vi "AutoAlign_P541.vi"() -> ()   [LabVIEW 2011]
uses:
  Controls/GraphNotifier2D.ctl
  Controls/StageStates.ctl
  <vilib>/LabVIEW Interface for Arduino/LabVIEW Interface for Arduino.lvlib
panel:
  out "Current Step":i32
  in  "Done":bool
  in  "Repeat":bool
  in  "Start":bool
  out "Cursor Position":dbl=40.46
  in  "InitialStep":dbl=-0.5
  in  "StepSize":dbl=0.03
  in  "Number Of Steps":i32=45
  out "Intensity Graph":sgl[][](graph)=[[1726.0, 1806.0, 1623.0, 1740.0, 1902.0, 2025.0, 2061.0, 2397.0, 1982.0, 2142.0, 1921.0, 1825.0, 1807.0, 1676.0, 1719.0], [1834.0, 1961.0, 1598.0, 2017.0, 2102.0, 2328.0, 2583.0, 2454.0, 2515.0, 2699.0, 2220.0, 2038.0, 1897.0, 1896.0, 1808.0], [1796.0, 1929.0, 2014.0, 2227.0, 2672.0, 3226.0, 3334.0, 3386.0, 3268.0, 2996.0, 2332.0, 2163.0, 1901.0, 1735.0, 1698.0], [1808.0, 2338.0, 2431.0, 2752.0, 3453.0, 4017.0, 4563.0, 4369.0, 4047.0, 3273.0, 2724.0, 2242.0, 2046.0, 1830.0, 1856.0], [1912.0, 2124.0, 3081.0, 2979.0, 5386.0, 11058.0, 13706.0, 11119.0, 6549.0, 3853.0, 2769.0, 2421.0, 1921.0, 1945.0, 1667.0], [1802.0, 2329.0, 2974.0, 5101.0, 13243.0, 29557.0, 37323.0, 29866.0, 11701.0, 4217.0, 2995.0, 2488.0, 2124.0, 2138.0, 1748.0], [1855.0, 2667.0, 2858.0, 6518.0, 22689.0, 47134.0, 57757.0, 40932.0, 16892.0, 4794.0, 2975.0, 2648.0, 2316.0, 1940.0, 2196.0], [1840.0, 2513.0, 2969.0, 6113.0, 20925.0, 44575.0, 52306.0, 35893.0, 13438.0, 3959.0, 2980.0, 2333.0, 2128.0, 1717.0, 1820.0], [1975.0, 2578.0, 2513.0, 4337.0, 10762.0, 22714.0, 27719.0, 17796.0, 6495.0, 3198.0, 2732.0, 2148.0, 1973.0, 1982.0, 1689.0], [1678.0, 2147.0, 2574.0, 2995.0, 4337.0, 7306.0, 8045.0, 5820.0, 3423.0, 2628.0, 2656.0, 2059.0, 2116.0, 1972.0, 1626.0], [1892.0, 2079.0, 2546.0, 2756.0, 2841.0, 3166.0, 3141.0, 2947.0, 2684.0, 2415.0, 1923.0, 1806.0, 2081.0, 1695.0, 1756.0], [1617.0, 1885.0, 1958.0, 2510.0, 2675.0, 2479.0, 2435.0, 2624.0, 2645.0, 2107.0, 1819.0, 2019.0, 1839.0, 1623.0, 1670.0], [1609.0, 1896.0, 1887.0, 1962.0, 2214.0, 2352.0, 2290.0, 2047.0, 1815.0, 2022.0, 1883.0, 1801.0, 1521.0, 1615.0, 1723.0], [1697.0, 1808.0, 1977.0, 1969.0, 2042.0, 1988.0, 2305.0, 2063.0, 1959.0, 1814.0, 1844.0, 1590.0, 1578.0, 1755.0, 1573.0], [1645.0, 1684.0, 1821.0, 1765.0, 1973.0, 1906.0, 2005.0, 1822.0, 1736.0, 1850.0, 1649.0, 1802.0, 1476.0, 1658.0, 1637.0]]
  in  "Quit":bool
  out "Sample":cluster{"X":dbl, "Y":dbl}[](graph)
  in  "Accumulations":i32=10
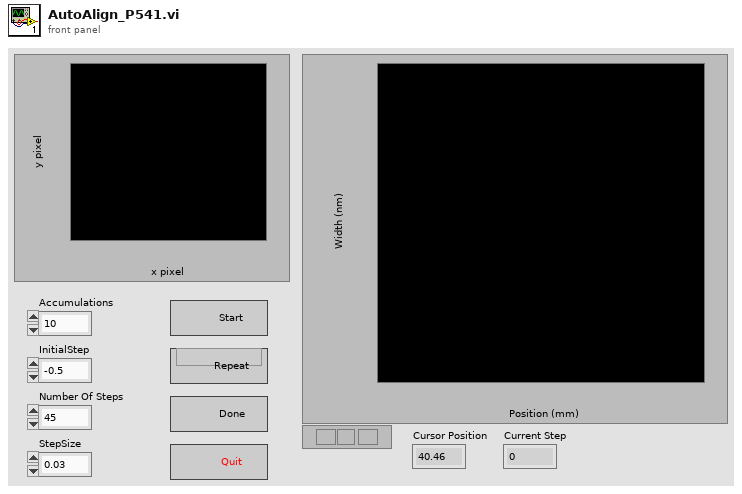
[diagram p1: front panel]
types:
  T1 = typedef "GraphNotifier2D.ctl" = cluster{"Xpos":i32, "Ypos":i32, "subarray":sgl[][], "Intensity":sgl}
  T2 = typedef "LabVIEW Interface for Arduino.lvlib/Arduino Resource.ctl" = cluster{"VISA resource":refnum<visa-resource-name>, "Board Type":T3, "Connection Type":enum8{"USB / Serial"}, "Bytes Per Packet (15)":u8}
  T3 = typedef "LabVIEW Interface for Arduino.lvlib/Board Type.ctl" = enum16{"Uno", "Dimuelanove w/Atmega 328", "Mega 2560"}
  T4 = typedef "StageStates.ctl" = enum16{"POSITION", "MVR", "MOVE", "HALT", "ONTARGET", "ERROR", "EXIT", "HOME", "ZEROPOS", "NANOPOS", "QUIT", "ANALOG"}
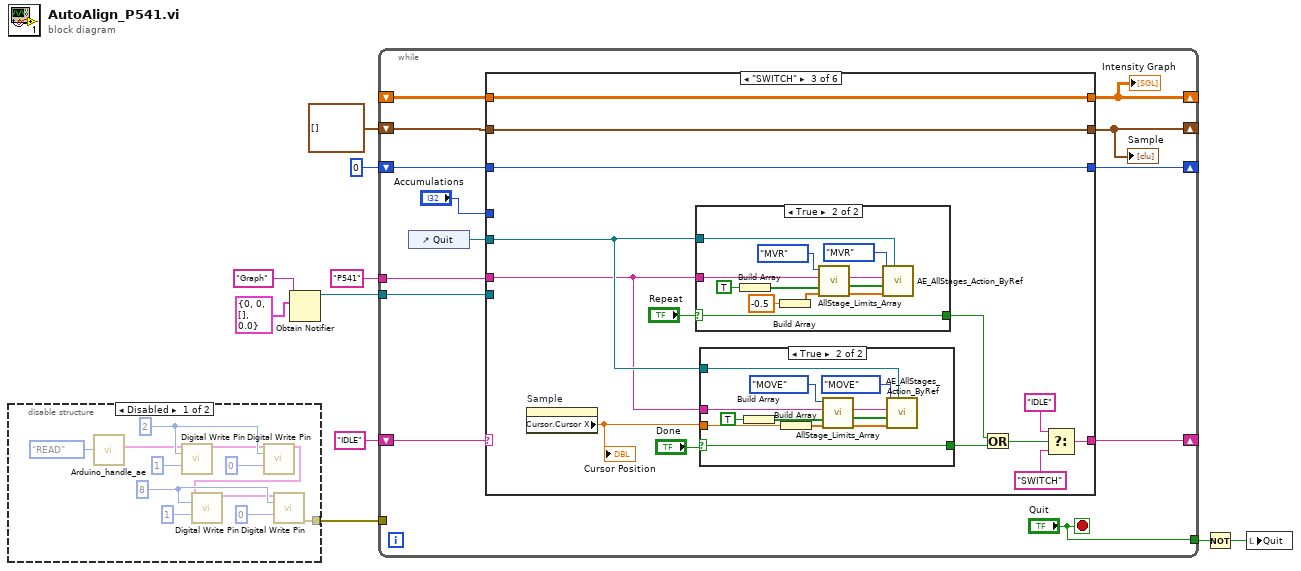
[diagram p0: block diagram]
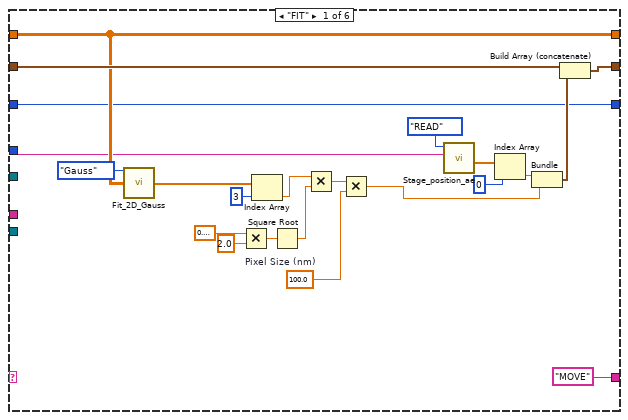
[diagram p3: hidden frame]
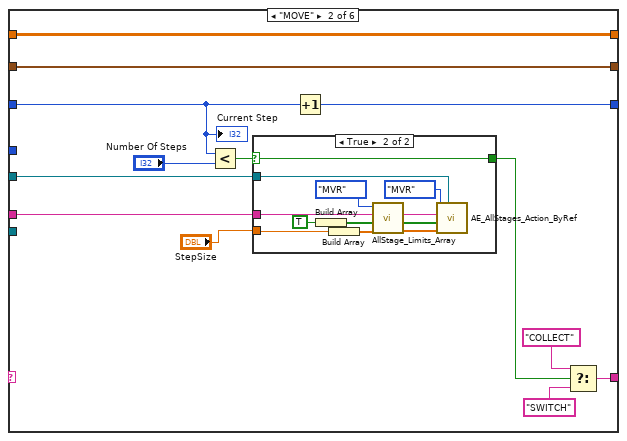
[diagram p4: hidden frame]
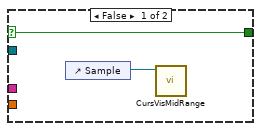
[diagram p5: hidden frame]
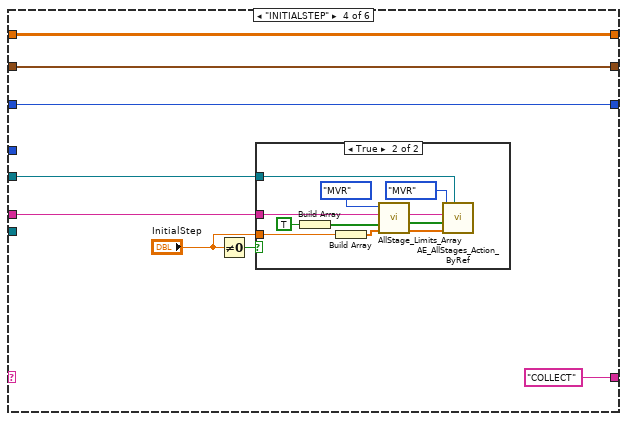
[diagram p8: hidden frame]
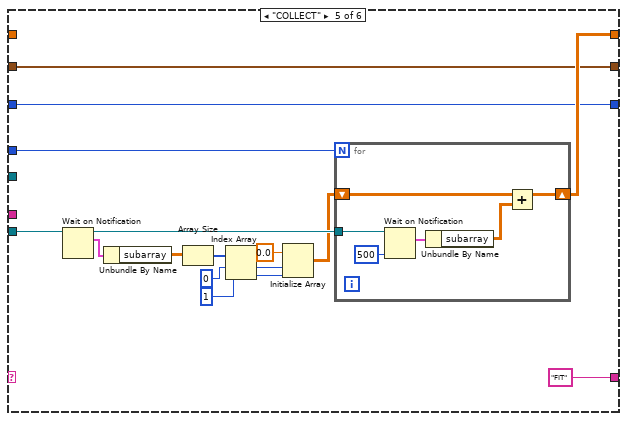
[diagram p10: hidden frame]
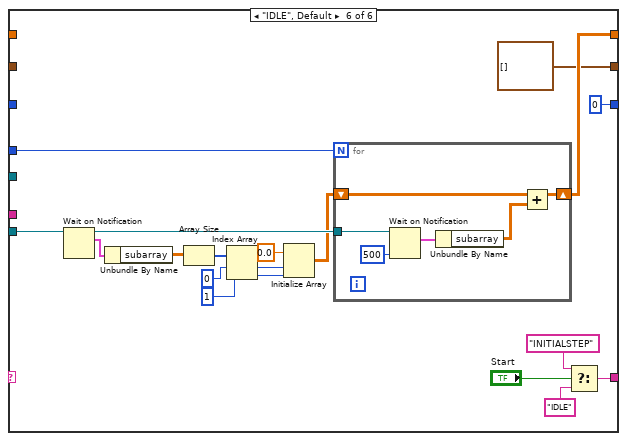
[diagram p11: hidden frame]
diagram:
  n1 = disable-structure shown="Disabled" {
    disable-tunnel: [w11 _] -> w6
    frame Disabled {
      w22 = u8 8 ("Digital I/O Pin (0)")
      w17 = u8 2 ("Digital I/O Pin (0)")
      n2 = call "Arduino_handle_ae.vi"("Enum"=enum16{"WRITE", "READ"}."READ") -> ("Arduino Resource Out"=w16:T2)  [unwired: 10 in]
      n3 = call <vilib>:"Digital Write Pin.vi"("Arduino Resource"=w16, "Digital I/O Pin (0)"=w17, "Value (0)"=u8 1) -> ("Arduino Resource"=w12:T2)  [unwired: 11 in, 1 out]
      n4 = call <vilib>:"Digital Write Pin.vi"("Arduino Resource"=w12, "Digital I/O Pin (0)"=w17, "Value (0)"=u8 0) -> ("Arduino Resource"=w21:T2)  [unwired: 11 in, 1 out]
      n5 = call <vilib>:"Digital Write Pin.vi"("Arduino Resource"=w21, "Digital I/O Pin (0)"=w22, "Value (0)"=u8 1) -> ("Arduino Resource"=w20:T2)  [unwired: 11 in, 1 out]
      n6 = call <vilib>:"Digital Write Pin.vi"("Arduino Resource"=w20, "Digital I/O Pin (0)"=w22, "Value (0)"=u8 0) -> ("error out"=w11:errorcluster)  [unwired: 11 in, 1 out]
    }
    frame Enabled {
    }
  }
  n7 = Obtain Notifier(name (unnamed)="Graph", notification data type=T1 {"Xpos"=0, "Ypos"=0, "subarray"=[], "Intensity"=0.0}) -> (notifier out=w3:refnum<notifier>)  [unwired: 2 in, 2 out]
  n8 = while {
    shift-right: [w33] -> _
    shift-left: _ -> [w35]
    shift-right: [w34] -> _
    shift-left: cluster{"x":dbl, "y":dbl}[] [] ("XY chart data") -> [w24]
    shift-right: [w32] -> _
    shift-left: "IDLE" -> [w28]
    shift-right: [w30] -> _
    shift-left: 0 ("NumberOfSteps 2") -> [w31]
    tunnel: w3 -> [w27]
    tunnel: "P541" ("StageID") -> [w25]
    tunnel: w6 -> [_]
    tunnel: ["Quit"] -> w2
    stop <- "Quit" stop-if-true
    n9 = control-ref of="Quit"() -> (w29:refnum<vi>)
    n10 = case shown="\"SWITCH\"" w28 {
      tunnel: [w53 w70 w96 w132 w159 w184] -> w33
      tunnel: w35 -> [w53 w70 w96 w132 _ _]
      tunnel: w24 -> [w55 w61 w97 w127 w158 _]
      tunnel: [w54 w61 w97 w127 w158 cluster{"x":dbl, "y":dbl}[] [] ("XY chart data")] -> w34
      tunnel: w25 -> [w50 w60 w93 w128 _ _]
      tunnel: ["MOVE" w67 w90 "COLLECT" "FIT" w182] -> w32
      tunnel: w31 -> [w51 w65 w98 w131 w157 _]
      tunnel: [w51 w66 w98 w131 w157 0 ("NumberOfSteps 2")] -> w30
      tunnel: w29 -> [_ w63 w95 w130 _ _]
      tunnel: w27 -> [_ _ _ _ w146 w175]
      tunnel: "Accumulations" -> [_ _ _ _ w155 w179]
      frame "FIT" {
        w42 = 100.0  # Pixel Size (nm)
        n11 = call "Fit_2D_Gauss.vi"("Enum"=enum16{"Gauss", "Lorentz"}."Gauss", "Image IN"=w53) -> ("Fit Parameters"=w57:dbl[])  [unwired: 12 in, 1 out]
        n12 = Multiply(x=0.6931471805599453, y=2.0) -> (x*y=w46:dbl)
        n13 = Index Array(array=w57, index=3) -> (element=w44:dbl)
        n14 = Square Root(x=w46) -> (sqrt(x)=w49:dbl)
        n15 = Multiply(x=w44, y=w49) -> (x*y=w45:dbl)
        n16 = Multiply(x=w45, y=w42) -> (x*y=w37:dbl)
        n17 = call "Stage_position_ae.vi"("StageID"=w50, "Enum"=enum16{"WRITE", "READ"}."READ") -> ("Position Out"=w40:dbl[])  [unwired: 8 in, 1 out]
        n18 = Index Array(array=w40, index=0) -> (element=w38:dbl)
        n19 = Bundle("Numeric"=w38, w37) -> (w56:cluster{"Numeric":dbl, dbl})  [unwired: 1 in]
        n20 = Build Array (concatenate)(w55, w56) -> (w54:cluster{"Numeric":dbl, "y":dbl}[])
      }
      frame "MOVE" {
        n21 = Less?(x=w65, y="Number Of Steps") -> (x < y?=w58:bool)
        n22 = case shown="True" w58 {
          selector: w58 -> [w72 w81]
          tunnel: w60 -> [_ w76]
          tunnel: w63 -> [_ w82]
          tunnel: [w72 w81] -> w64
          tunnel: "StepSize" -> [_ w74]
          frame False {
            n23 = control-ref of="Sample"() -> (w71:refnum<vi>)
            n24 = call "CursVisMidRange.vi"("XYGraph in"=w71) -> ()  [unwired: 11 in]
          }
          frame True {
            n25 = Build Array(TRUE) -> (w77:bool[])
            n26 = Build Array(w74) -> (w73:dbl[])
            n27 = call "AllStage_Limits_Array.vi"("Step(um)/Position(units)"=w73, "Axis"=w77, "Stage ID"=w76, "MOVE/MVR"=enum16{"MOVE", "MVR"}."MVR") -> ("Positions"=w78:dbl[], "Boolean Array"=w79:bool[], "Stage ID"=w80:string)  [unwired: 5 in]
            n28 = call "AE_AllStages_Action_ByRef.vi"("Abort"=w82, "Positions"=w78, "Axis"=w79, "Stage ID"=w80, "Action"=StageStates."MVR") -> ()  [unwired: 3 in, 4 out]
          }
        }
        n29 = Increment(x=w65) -> (x+1=w66:i32)
        n30 = Select(t="COLLECT", s=w64, f="SWITCH") -> (s? t:f=w67:string)
        "Current Step" <- w65
      }
      frame "SWITCH" {
        n31 = property on="Sample" class="XYGraph (strict)"() -> ("Cursor.Cursor X"=w94:dbl)  [unwired: 2 in, 2 out]
        "Cursor Position" <- w94
        n32 = case shown="True" "Repeat" {
          selector: "Repeat" -> [w112 w114]
          tunnel: w93 -> [_ w115]
          tunnel: w95 -> [_ w122]
          tunnel: [w112 w114] -> w86
          frame False {
          }
          frame True {
            n33 = Build Array(TRUE) -> (w120:bool[])
            n34 = Build Array(-0.5 ("Step(um)/Position(units)")) -> (w113:dbl[])
            n35 = call "AllStage_Limits_Array.vi"("Step(um)/Position(units)"=w113, "Axis"=w120, "Stage ID"=w115, "MOVE/MVR"=enum16{"MOVE", "MVR"}."MVR") -> ("Positions"=w117:dbl[], "Boolean Array"=w118:bool[], "Stage ID"=w119:string)  [unwired: 5 in]
            n36 = call "AE_AllStages_Action_ByRef.vi"("Abort"=w122, "Positions"=w117, "Axis"=w118, "Stage ID"=w119, "Action"=StageStates."MVR") -> ()  [unwired: 3 in, 4 out]
          }
        }
        n37 = case shown="True" "Done" {
          selector: "Done" -> [w99 w101]
          tunnel: w93 -> [_ w102]
          tunnel: w95 -> [_ w109]
          tunnel: w94 -> [_ w103]
          tunnel: [w99 w101] -> w85
          frame False {
          }
          frame True {
            n38 = Build Array(TRUE) -> (w107:bool[])
            n39 = Build Array(w103) -> (w100:dbl[])
            n40 = call "AllStage_Limits_Array.vi"("Step(um)/Position(units)"=w100, "Axis"=w107, "Stage ID"=w102, "MOVE/MVR"=enum16{"MOVE", "MVR"}."MOVE") -> ("Positions"=w104:dbl[], "Boolean Array"=w105:bool[], "Stage ID"=w106:string)  [unwired: 5 in]
            n41 = call "AE_AllStages_Action_ByRef.vi"("Abort"=w109, "Positions"=w104, "Axis"=w105, "Stage ID"=w106, "Action"=StageStates."MOVE") -> ()  [unwired: 3 in, 4 out]
          }
        }
        n42 = Or(x=w86, y=w85) -> (x .or. y?=w89:bool)
        n43 = Select(t="IDLE", s=w89, f="SWITCH") -> (s? t:f=w90:string)
      }
      frame "INITIALSTEP" {
        n44 = Not Equal To 0?(x="InitialStep") -> (x != 0?=w126:bool)
        n45 = case shown="True" w126 {
          tunnel: w128 -> [_ w139]
          tunnel: w130 -> [_ w141]
          tunnel: "InitialStep" -> [_ w140]
          frame False {
          }
          frame True {
            n46 = Build Array(TRUE) -> (w137:bool[])
            n47 = Build Array(w140) -> (w133:dbl[])
            n48 = call "AllStage_Limits_Array.vi"("Step(um)/Position(units)"=w133, "Axis"=w137, "Stage ID"=w139, "MOVE/MVR"=enum16{"MOVE", "MVR"}."MVR") -> ("Positions"=w134:dbl[], "Boolean Array"=w135:bool[], "Stage ID"=w136:string)  [unwired: 5 in]
            n49 = call "AE_AllStages_Action_ByRef.vi"("Abort"=w141, "Positions"=w134, "Axis"=w135, "Stage ID"=w136, "Action"=StageStates."MVR") -> ()  [unwired: 3 in, 4 out]
          }
        }
      }
      frame "COLLECT" {
        n50 = Wait on Notification(notifier=w146) -> (notifier out=w145:refnum<notifier>, notification=w154:T1)  [unwired: 3 in, 2 out]
        n51 = Unbundle By Name(w154) -> ("subarray"=w153:sgl[][])
        n52 = Array Size(array=w153) -> (size(s)=w152:i32[])
        n53 = Index Array(array=w152, index #1=0 ("index"), index #2=1 ("index")) -> (element #1=w149:i32, element #2=w148:i32)
        n54 = Initialize Array(sgl 0.0 ("element"), w149, w148) -> (w144:sgl[][])
        n55 = for {
          N: w155 -> [_]
          shift-right: [w165] -> w159
          shift-left: w144 -> [w164]
          tunnel: w145 -> [w162]
          n56 = Wait on Notification(notifier=w162, timeout in ms (-1)=500) -> (notification=w161:T1)  [unwired: 2 in, 3 out]
          n57 = Unbundle By Name(w161) -> ("subarray"=w160:sgl[][])
          n58 = Add(x=w164, y=w160) -> (x+y=w165:sgl[][])
        }
      }
      frame "IDLE", Default {
        n59 = Wait on Notification(notifier=w175) -> (notifier out=w174:refnum<notifier>, notification=w177:T1)  [unwired: 3 in, 2 out]
        n60 = Unbundle By Name(w177) -> ("subarray"=w176:sgl[][])
        n61 = Array Size(array=w176) -> (size(s)=w173:i32[])
        n62 = Index Array(array=w173, index #1=0 ("index"), index #2=1 ("index")) -> (element #1=w170:i32, element #2=w169:i32)
        n63 = Initialize Array(sgl 0.0 ("element"), w170, w169) -> (w167:sgl[][])
        n64 = for {
          N: w179 -> [_]
          shift-right: [w190] -> w184
          shift-left: w167 -> [w189]
          tunnel: w174 -> [w187]
          n65 = Wait on Notification(notifier=w187, timeout in ms (-1)=500) -> (notification=w186:T1)  [unwired: 2 in, 3 out]
          n66 = Unbundle By Name(w186) -> ("subarray"=w185:sgl[][])
          n67 = Add(x=w189, y=w185) -> (x+y=w190:sgl[][])
        }
        n68 = Select(t="INITIALSTEP", s="Start", f="IDLE") -> (s? t:f=w182:string)
      }
    }
    "Sample" <- w34
    "Intensity Graph" <- w33
  }
  n69 = Not(x=w2) -> (.not. x?=w1:bool)
  n70 = local write "Quit"(w1) -> ()
